vi "base format to strings.vi"(8 "error in":errorcluster, 11 "format":T5) -> (0 "error out":errorcluster, 3 "data":T1)   [LabVIEW 2023, in "CEF.lvlib"]
doc: "Convert the lowest level file format (version+data) into the lowest-level structured memory format, in this case (1.0.0) a set of flattened instance data.Copyright 2017 National Instruments Corporation\n\nLicensed under the Apache License, Version 2.0 (the \"License\"); you may not use this file except in compliance with the License. You may obtain a copy of the License at http://www.apache.org/licenses/LICENSE-2.0\nUnless required by applicable law or agreed to in writing, software distributed under the License is distributed on an \"AS IS\" BASIS, WITHOUT WARRANTIES OR CONDITIONS OF ANY KIND, either express or implied. See the License for the specific language governing permissions and limitations under the License."
uses:
  CEF.lvlib
  base file format.ctl
  flat hierarchy.ctl
  hierarchy repo/full hierarchy.ctl
  hierarchy element.ctl
  instance data.ctl
  hierarchy repo/CEF_HierarchyRepo.lvclass
  serializable configuration/CEF_serializable configuration.lvclass
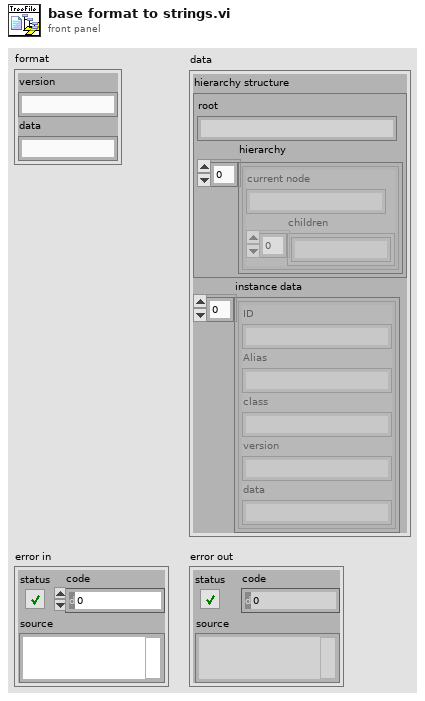
[diagram p1: front panel]
types:
  T1 = typedef "CEF.lvlib/flat hierarchy.ctl" = cluster{"hierarchy structure":T2, "instance data":T4[]}
  T2 = typedef "CEF.lvlib/CEF_HierarchyRepo.lvclass/full hierarchy.ctl" = cluster{"root":string, "hierarchy":T3[]}
  T3 = typedef "CEF.lvlib/hierarchy element.ctl" = cluster{"current node":string, "children":string[]}
  T4 = typedef "CEF.lvlib/instance data.ctl" = cluster{"ID":string, "Alias":string, "class":string, "version":string, "data":string}
  T5 = typedef "CEF.lvlib/base file format.ctl" = cluster{"version":string, "data":string}
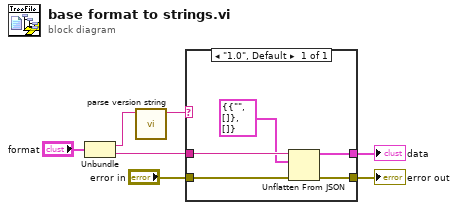
[diagram p0: block diagram]
diagram:
  n1 = Unbundle("format") -> ("version"=w6:string, "data"=w4:string)
  n2 = call "parse version string.vi"("full version"=w6) -> ("major.minor version"=w5:string)  [unwired: 7 in, 3 out]
  n3 = case shown="\"1.0\", Default" w5 {
    tunnel: w4 -> [w10]
    tunnel: [w12] -> w3
    tunnel: "error in" -> [w11]
    tunnel: [w8] -> w1
    frame "1.0", Default {
      n4 = Unflatten From JSON(JSON string=w10, type and defaults=T1 {"hierarchy structure"={"root"="", "hierarchy"=[]}, "instance data"=[]} ("1.0.0"), error in (no error)=w11) -> (value=w8:T1, error out=w12:errorcluster)  [unwired: 4 in]
    }
  }
  "error out" <- w3
  "data" <- w1
